vi "View.vi"(8 "error in (no error)":errorcluster, 11 "Worker In":refnum<class "Worker.lvclass">) -> (0 "error out":errorcluster, 3 "Worker Out":refnum<class "Worker.lvclass">)   [LabVIEW 2020, in "Worker.lvclass"]
doc: "This VI implements the main UI of the process. A reference to this VI should be set using the Set View VI Reference.vi method when the VI is started."
uses:
  Worker.lvclass
  C:/Program Files (x86)/National Instruments/LabVIEW 2020/vi.lib/Asteme/Triarc Framework/Process/Process.lvclass
  C:/Program Files (x86)/National Instruments/LabVIEW 2020/vi.lib/Asteme/Triarc Framework/View/View.lvclass
  <vilib>/Asteme/Triarc Framework/View/View.lvclass/View.ctl
  <vilib>/Asteme/Triarc Framework/View/View.lvclass
  <vilib>/Asteme/Triarc Framework/Process/Process.lvclass
panel:
  out "Name":string
  out "Worker Type":string="Barista"
  out "Orders Filled This Shift":u32
  out "Status":string="Waiting..."
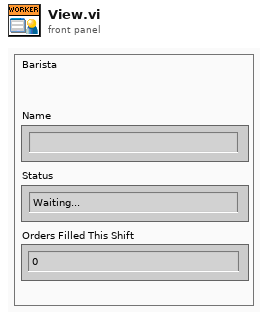
[diagram p1: front panel]
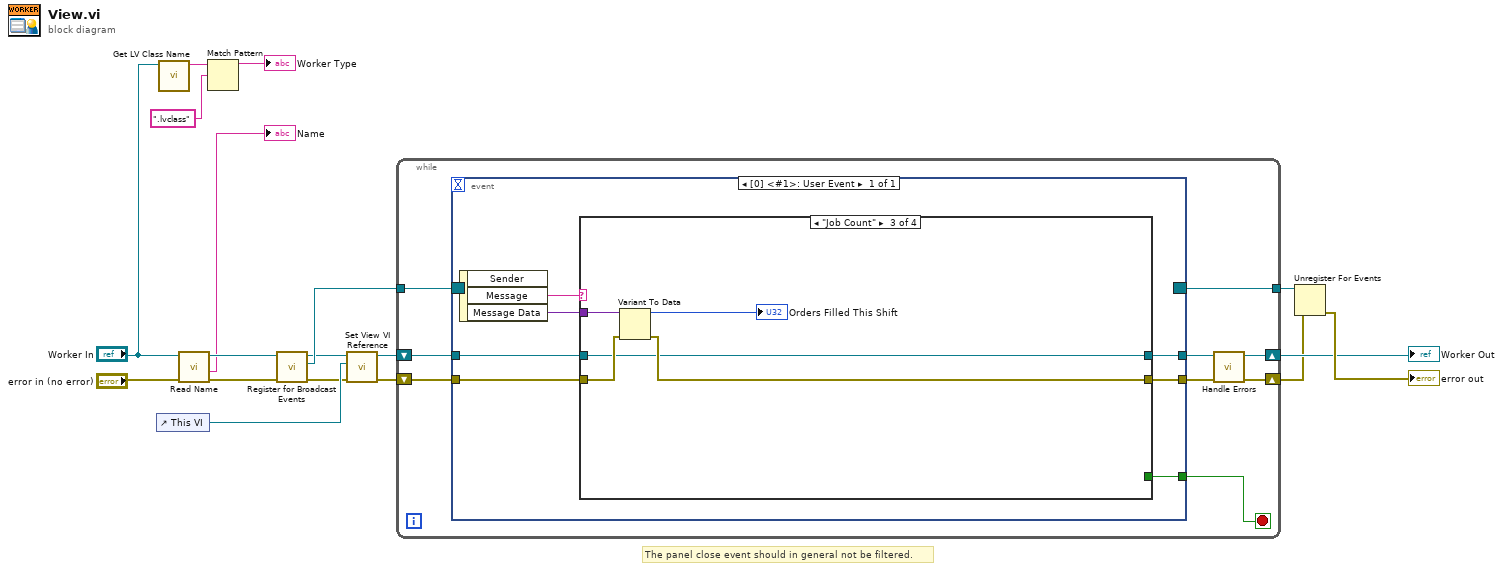
[diagram p0: block diagram]
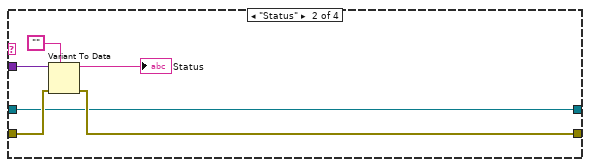
[diagram p3: hidden frame]
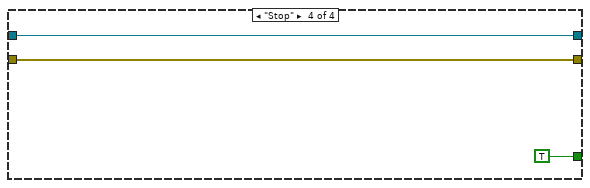
[diagram p4: hidden frame]
diagram:
  # "The panel close event should in general not be filtered."
  n1 = control-ref of="This VI"() -> (w16:refnum<vi>)
  n2 = call <vilib>:"Get LV Class Name.vi"("object"="Worker In") -> ("class name"=w8:string)  [unwired: 9 in, 1 out]
  n3 = call-dynamic "Read Name.vi"("error in (no error)"="error in (no error)", "Process In"="Worker In") -> ("error out"=w4:errorcluster, "Name"=→"Name":string, "Process Out"=w2:refnum<class "Worker.lvclass">)  [unwired: 6 in, 1 out]
  n4 = Match Pattern(string=w8, regular expression=".lvclass") -> (before substring=→"Worker Type":string)  [unwired: 1 in, 3 out]
  n5 = call <vilib>:"Register for Broadcast Events.vi"("error in (no error)"=w4, "Process In"=w2) -> ("error out"=w14:errorcluster, "Event Registration Refnum Out"=w15:refnum<event-registration>, "Process Out"=w13:refnum<class "Worker.lvclass">)  [unwired: 7 in]
  n6 = call <vilib>:"Set View VI Reference.vi"("error in (no error)"=w14, "View VI Reference"=w16, "UI View in"=w13) -> ("error out"=w12:errorcluster, "UI View out"=w11:refnum<class "Worker.lvclass">)  [unwired: 7 in]
  n7 = while {
    shift-right: [w21] -> w17
    shift-left: w11 -> [w27]
    shift-right: [w19] -> w10
    shift-left: w12 -> [w25]
    tunnel: w15 -> [w24]
    tunnel: [w23] -> w9
    stop <- w22 stop-if-true
    n8 = event shown="[0] <#1>: User Event" {
      selector: w24 -> [_]
      dyn-events: [_] -> w23
      timeout: _ -> [_]
      tunnel: w27 -> [w34]
      tunnel: [w33] -> w26
      tunnel: w25 -> [w31]
      tunnel: [w32] -> w20
      tunnel: [w29] -> w22
      event User Event {
        n9 = event-data() -> ("Message"=w30:string, "Message Data"=w28:variant)  [unwired: 1 in, 1 out]
        n10 = case shown="\"Job Count\"" w30 {
          tunnel: w34 -> [w36 w37 w44 w50]
          tunnel: [w36 w37 w44 w50] -> w33
          tunnel: [w35 w38 w45 w49] -> w32
          tunnel: w31 -> [w35 w41 w46 w49]
          tunnel: [_ _ _ TRUE] -> w29
          tunnel: w28 -> [_ w42 w47 _]
          frame Default {
          }
          frame "Status" {
            n11 = Variant To Data(error in=w41, type="", Variant=w42) -> (data=→"Status":string, error out=w38:errorcluster)
          }
          frame "Job Count" {
            n12 = Variant To Data(error in=w46, Variant=w47) -> (data=→"Orders Filled This Shift":u32, error out=w45:errorcluster)  [unwired: 1 in]
          }
          frame "Stop" {
          }
        }
      }
    }
    n13 = call-dynamic "Handle Errors.vi"("error in (no error)"=w20, "Process In"=w26) -> ("error out"=w19:errorcluster, "Process Out"=w21:refnum<class "Worker.lvclass">)  [unwired: 8 in]
  }
  "Worker Out" <- w17
  n14 = Unregister For Events(event registration refnum=w9, error in=w10) -> (error out=→"error out":errorcluster)
